vi "check_option.vi"(5 "Error generation (Error if missing)":T1, 7 "Attribute":T2={"Identifier"="", "Descriptive Name"="", "Data Type"=enum."Integer 32", "Command"="", "Access"=enum."Read/Write", "Range Table"="", "Read Callback"="", "Write Callback"="", "Supported Models"="", "Instrument Options"="", "Index"=0, "OPC Wait"=FALSE, "No Status Check"=FALSE, "Cache Only"=FALSE}, 8 "error in":errorcluster caption="error in (no error)", 11 "VISA resource name":refnum<visa-resource-name>) -> (0 "error out":errorcluster, 2 "Option installed":bool, 3 "VISA resource name out":refnum<visa-resource-name>)   [LabVIEW 2022 SP3, in "hmp4000_rsidr_core.lvlib"]
uses:
  hmp4000_rsidr_core.lvlib
  type_Attribute.ctl
  type_Attribute_Data_Type.ctl
  type_ReadWriteAccess.ctl
  type_InstrOptions_Error_GenMode.ctl
  type_Error_Codes.ctl
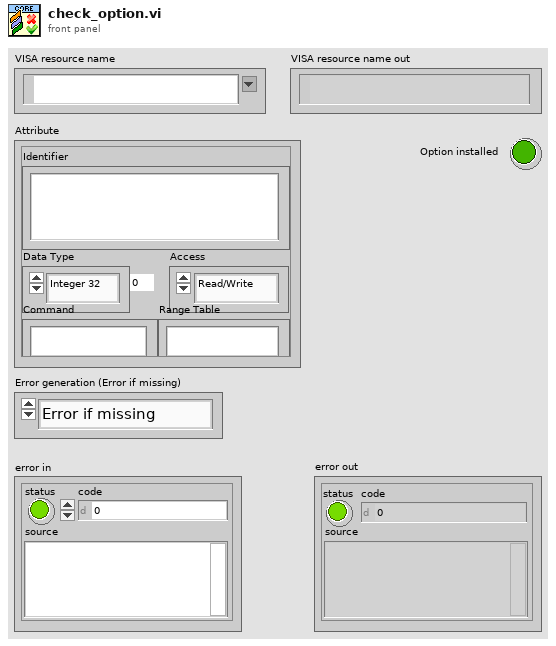
[diagram p1: front panel]
types:
  T1 = typedef "hmp4000_rsidr_core.lvlib/type_InstrOptions_Error_GenMode.ctl" = enum16{"Error if missing", "Error if present", "No error"}
  T2 = typedef "hmp4000_rsidr_core.lvlib/type_Attribute.ctl" = cluster{"Identifier":string, "Descriptive Name":string, "Data Type":T3, "Command":string, "Access":T4, "Range Table":string, "Read Callback":string, "Write Callback":string, "Supported Models":string, "Instrument Options":string, "Index":i32, "OPC Wait":bool, "No Status Check":bool, "Cache Only":bool}
  T3 = typedef "hmp4000_rsidr_core.lvlib/type_Attribute_Data_Type.ctl" = enum16{"Integer 32", "Double", "String", "Boolean", "None", "Integer 64", "RawString"}
  T4 = typedef "hmp4000_rsidr_core.lvlib/type_ReadWriteAccess.ctl" = enum16{"Read Only", "Write Only", "Read/Write"}
  T5 = typedef "hmp4000_rsidr_core.lvlib/type_Error_Codes.ctl" = enum16{"No_error", "VISA_err_ResourceNotFound", "VISA_err_Timeout", "VISA_warn_MoreDataAvailable", "RS_err_MissingCallback", "RS_err_InvalidAttribute", "RS_err_InvalidValue", "RS_err_UnknownResource", "RS_err_AlreadyInitialized", "RS_err_InstrumentStatus", "RS_err_BadRepCapName", "RS_err_TypesMismatch", "RS_err_ValueNotSupported", "RS_err_InvalidRngTable", "RS_err_IDqueryFail", "RS_err_UnexpResponse", "VISA_warn_ConfigNotLoaded", "RS_err_AttributeNotReadable", "RS_err_AttributeNotWritable", "RS_err_InstrumentType", "RS_err_InstrumentOption", "VISA_err_InvalidSize", "RS_err_ReliabilityIndicator", "VISA_warn_UnknownStatus", "VISA_warn_TermCharRead", "VISA_err_IO_error", "RS_err_FunctionNotSupported", "VISA_warn_QueueEmpty"}
  T6 = typedef "hmp4000_rsidr_core.lvlib/type_Session_Data.ctl" = cluster{"IDN string":string, "Instrument FW":string, "Instr type":string, "Instr type for err. msg.":string, "Installed Options":string[], "Ignore Error Messages":string, "Logging params":variant, "OPC Timeout":i32, "VISA Timeout":i32, "STB Poll VISA Timeout":i32, "Additional Flags":i32, "Wait Before Read":i32, "Wait Before Write":i32, "Option String Flags":i32, "IO Segment Size":i64, "VISA Access Mode":T7, "Interface Type":T8, "OPC Wait Mode":T9, "Bin Float Number  Format":T10, "Bin Integer Number Format":T11, "Simulate":bool, "VXIcapable":bool, "Duplicate Session":bool, "Add LF to Write":bool, "Logging":bool, "Fast Sweep":bool, "Query Instrument Status":bool, "Check Range":bool, "Check Options":bool}
  T7 = typedef "hmp4000_rsidr_core.lvlib/type_VisaAccessMode.ctl" = u16
  T8 = typedef "hmp4000_rsidr_core.lvlib/type_InterfaceType.ctl" = enum16{"Unknown", "GPIB", "VXI", "GPIB_VXI", "ASRL", "PXI", "TCPIP", "USB", "SOCKET"}
  T9 = typedef "hmp4000_rsidr_core.lvlib/type_OPC_Wait_Mode.ctl" = enum16{"STBpolling", "STBpollingSlow", "STBpollingSuperSlow", "ServiceRequest", "OPCquery"}
  T10 = typedef "hmp4000_rsidr_core.lvlib/type_Binary_Float_Number_Format.ctl" = enum16{"Float_4_Bytes_Swapped", "Float_4_Bytes", "Double_8_Bytes_Swapped", "Double_8_Bytes"}
  T11 = typedef "hmp4000_rsidr_core.lvlib/type_Binary_Integer_Number_Format.ctl" = enum16{"Int32_4_Bytes_Swapped", "Int32_4 Bytes", "Int16_2_Bytes_Swapped", "Int16_2_Bytes"}
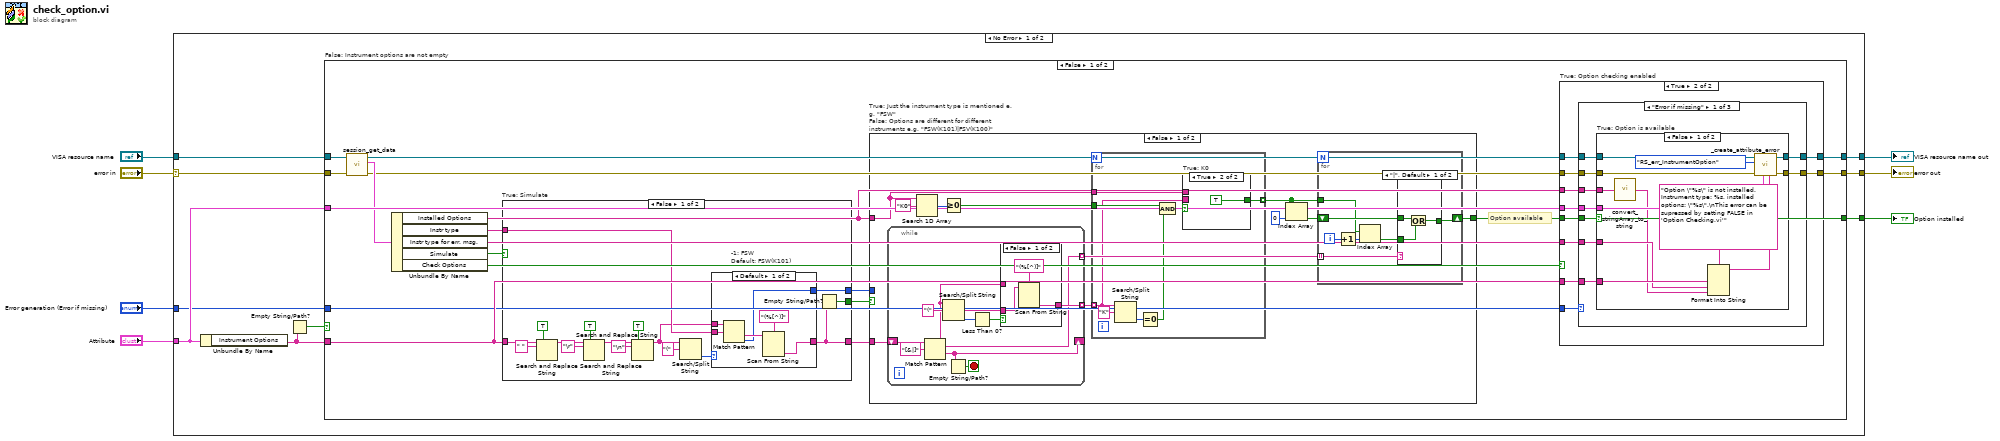
[diagram p0: block diagram]
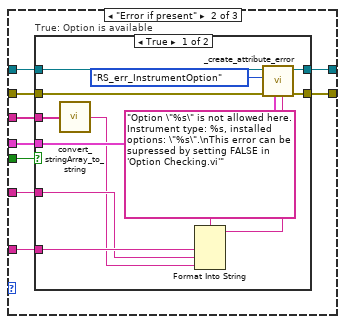
[diagram p4: hidden frame]
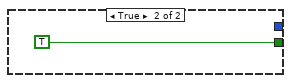
[diagram p8: hidden frame]
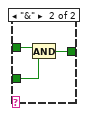
[diagram p9: hidden frame]
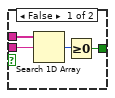
[diagram p10: hidden frame]
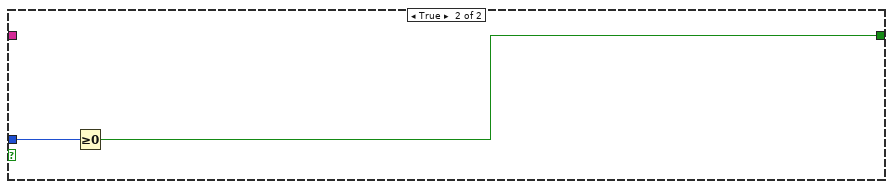
[diagram p12: hidden frame]
diagram:
  n1 = case shown="No Error" "error in" {
    selector: "error in" -> [w11 w176]
    tunnel: [w16 w176] -> w7
    tunnel: "Attribute" -> [w15 _]
    tunnel: "VISA resource name" -> [w10 w177]
    tunnel: [w13 w177] -> w4
    tunnel: "Error generation (Error if missing)" -> [w8 _]
    tunnel: [w9 _] -> w1
    frame No Error {
      n2 = Unbundle By Name(w15) -> ("Instrument Options"=w14:string)
      n3 = Empty String/Path?(string/path=w14) -> (empty?=w12:bool)
      n4 = case "False: Instrument options are not empty" shown="False" w12 {
        tunnel: w11 -> [w24 w175]
        tunnel: [w35 w175] -> w16
        tunnel: w14 -> [w32 _]
        tunnel: w15 -> [w33 _]
        tunnel: w10 -> [w23 w174]
        tunnel: [w27 w174] -> w13
        tunnel: [w17 _] -> w9
        tunnel: w8 -> [w19 _]
        frame False {
          # "Option available"
          n5 = call "session_get_data.vi"("error in"=w24, "VISA resource name"=w23) -> ("error out"=w21:errorcluster, "Session User Data out"=w22:T6, "VISA resource name out"=w20:refnum<visa-resource-name>)  [unwired: 6 in, 1 out]
          n6 = Unbundle By Name(w22) -> ("Installed Options"=w26:string[], "Instr type"=w34:string, "Instr type for err. msg."=w31:string, "Simulate"=w25:bool, "Check Options"=w18:bool)
          n7 = case "True: Simulate" shown="False" w25 {
            tunnel: w34 -> [w111 _]
            tunnel: w32 -> [w110 _]
            tunnel: [w98 _] -> w30
            tunnel: [w96 TRUE] -> w29
            tunnel: [w97 _] -> w28
            frame False {
              n8 = Search and Replace String(replace all?=TRUE ("replace all? (F)"), input string=w110, search string=" ") -> (result string=w103:string)  [unwired: 5 in, 3 out]
              n9 = Search and Replace String(replace all?=TRUE ("replace all? (F)"), input string=w103, search string="\r") -> (result string=w102:string)  [unwired: 5 in, 3 out]
              n10 = Search and Replace String(replace all?=TRUE ("replace all? (F)"), input string=w102, search string="\n") -> (result string=w99:string)  [unwired: 5 in, 3 out]
              n11 = Search/Split String(string=w99, search string/char (-)="(") -> (offset of match=w100:i32)  [unwired: 1 in, 2 out]
              n12 = case "-1: FSW\nDefault: FSW(K101)" shown="Default" w100 {
                tunnel: w99 -> [w117 w118]
                tunnel: [w113 w118] -> w97
                tunnel: w111 -> [w116 _]
                tunnel: [w112 _] -> w98
                frame Default {
                  n13 = Match Pattern(string=w117, regular expression=w116) -> (after substring=w115:string, offset past match=w112:i32)  [unwired: 1 in, 2 out]
                  n14 = Scan From String(format string="(%[^)]", input string=w115) -> (output 1=w113:string)  [unwired: 3 in, 3 out]
                }
                frame -1 {
                }
              }
              n15 = Empty String/Path?(string/path=w97) -> (empty?=w96:bool)
            }
            frame True {
            }
          }
          n16 = case "True: Just the instrument type is mentioned e.g. \"FSW\"\nFalse: Options are different for different instruments e.g. \"FSW(K101)|FSV(K100)\"" shown="False" w29 {
            tunnel: [w127 w172] -> w17
            tunnel: w28 -> [w126 _]
            tunnel: w26 -> [w124 _]
            tunnel: w30 -> [_ w173]
            frame False {
              n17 = while {
                shift-right: [w157] -> _
                shift-left: w126 -> [w167]
                tunnel: [w160] -> w120 mode=indexing
                tunnel: [w159] -> w130 mode=indexing
                stop <- w165 stop-if-true
                n18 = Match Pattern(string=w167, regular expression="[&|]") -> (before substring=w158:string, match substring=w159:string, after substring=w157:string)  [unwired: 1 in, 1 out]
                n19 = Search/Split String(string=w158, search string/char (-)="(") -> (match + rest of string=w163:string, offset of match=w162:i32)  [unwired: 1 in, 1 out]
                n20 = Empty String/Path?(string/path=w157) -> (empty?=w165:bool)
                n21 = Less Than 0?(x=w162) -> (x < 0?=w161:bool)
                n22 = case shown="False" w161 {
                  tunnel: w163 -> [w168 _]
                  tunnel: [w169 w171] -> w160
                  tunnel: w158 -> [_ w171]
                  frame False {
                    n23 = Scan From String(format string="(%[^)]", input string=w168) -> (output 1=w169:string)  [unwired: 3 in, 3 out]
                  }
                  frame True {
                  }
                }
              }
              n24 = Search 1D Array(1D array=w124, element="K0") -> (index of element=w122:i32)  [unwired: 1 in]
              n25 = Greater Or Equal To 0?(x=w122) -> (x >= 0?=w121:bool)
              n26 = for {
                tunnel: w124 -> [w151]
                tunnel: [w150] -> w125 mode=indexing
                tunnel: w121 -> [w146]
                tunnel: w120 -> [w145] mode=indexing
                n27 = Search/Split String(string=w145, search string/char (-)="K") -> (offset of match=w148:i32)  [unwired: 1 in, 2 out]
                n28 = Equal To 0?(x=w148) -> (x = 0?=w147:bool)
                n29 = Compound Arithmetic op=AND(w146, w147) -> (w144:bool)
                n30 = case "True: K0" shown="True" w144 {
                  tunnel: w151 -> [w155 _]
                  tunnel: [w153 TRUE] -> w150
                  tunnel: w145 -> [w152 _]
                  frame False {
                    n31 = Search 1D Array(1D array=w155, element=w152) -> (index of element=w154:i32)  [unwired: 1 in]
                    n32 = Greater Or Equal To 0?(x=w154) -> (x >= 0?=w153:bool)
                  }
                  frame True {
                  }
                }
              }
              n33 = Index Array(array=w125, index=0) -> (element=w129:bool)
              n34 = for {
                tunnel: w130 -> [w131] mode=indexing
                tunnel: w125 -> [w135]
                shift-right: [w136] -> w127
                shift-left: w129 -> [w137]
                i -> [w133]
                n35 = Increment(x=w133) -> (x+1=w134:i32)
                n36 = Index Array(array=w135, index=w134) -> (element=w132:bool)
                n37 = case shown="\"|\", Default" w131 {
                  tunnel: w137 -> [w139 w143]
                  tunnel: [w140 w142] -> w136
                  tunnel: w132 -> [w138 w141]
                  frame "|", Default {
                    n38 = Or(x=w139, y=w138) -> (x .or. y?=w140:bool)
                  }
                  frame "&" {
                    n39 = And(x=w143, y=w141) -> (x .and. y?=w142:bool)
                  }
                }
              }
            }
            frame True {
              n40 = Greater Or Equal To 0?(x=w173) -> (x >= 0?=w172:bool)
            }
          }
          n41 = case "True: Option checking enabled" shown="True" w18 {
            tunnel: [w37 w47] -> w35
            tunnel: w33 -> [_ w46]
            tunnel: w32 -> [_ w45]
            tunnel: w31 -> [_ w44]
            tunnel: [w36 w43] -> w27
            tunnel: w26 -> [_ w42]
            tunnel: w21 -> [w37 w41]
            tunnel: w20 -> [w36 w40]
            tunnel: w19 -> [_ w39]
            tunnel: w17 -> [_ w38]
            frame False {
            }
            frame True {
              n42 = case shown="\"Error if missing\"" w39 {
                tunnel: [w56 w79 w95] -> w47
                tunnel: w46 -> [w55 w78 _]
                tunnel: w45 -> [w54 w77 _]
                tunnel: w44 -> [w53 w76 _]
                tunnel: [w52 w75 w94] -> w43
                tunnel: w42 -> [w51 w74 _]
                tunnel: w41 -> [w50 w73 w95]
                tunnel: w40 -> [w49 w72 w94]
                tunnel: w38 -> [w48 w71 _]
                frame "Error if missing" {
                  n43 = case "True: Option is available" shown="False" w48 {
                    tunnel: w50 -> [w67 w70]
                    tunnel: [w68 w70] -> w56
                    tunnel: w55 -> [w64 _]
                    tunnel: w54 -> [w66 _]
                    tunnel: w53 -> [w58 _]
                    tunnel: w49 -> [w61 w69]
                    tunnel: [w60 w69] -> w52
                    tunnel: w51 -> [w59 _]
                    frame False {
                      n44 = call "convert_stringArray_to_string.vi"("string array in"=w59) -> ("string out"=w57:string)  [unwired: 4 in]
                      n45 = Format Into String(format string="Option \"%s\" is not installed. Instrument type: %s, installed options: \"%s\".\nThis error can be supressed by setting FALSE in 'Option Checking.vi'" ("string"), w66, w58, w57) -> (resulting string=w63:string)  [unwired: 2 in, 1 out]
                      n46 = call "_create_attribute_error.vi"("Error Elaboration (\"\")"=w63, "Attribute"=w64, "error in"=w67, "Error Enum in"=type_Error_Codes."RS_err_InstrumentOption" ("Error Enum in (from err to recompose)"), "VISA resource name"=w61) -> ("error out"=w68:errorcluster, "VISA resource name out"=w60:refnum<visa-resource-name>)  [unwired: 5 in]
                    }
                    frame True {
                    }
                  }
                }
                frame "Error if present" {
                  n47 = case "True: Option is available" shown="True" w71 {
                    tunnel: w73 -> [w90 w93]
                    tunnel: [w91 w93] -> w79
                    tunnel: w78 -> [w87 _]
                    tunnel: w77 -> [w89 _]
                    tunnel: w76 -> [w81 _]
                    tunnel: w72 -> [w84 w92]
                    tunnel: [w83 w92] -> w75
                    tunnel: w74 -> [w82 _]
                    frame True {
                      n48 = call "convert_stringArray_to_string.vi"("string array in"=w82) -> ("string out"=w80:string)  [unwired: 4 in]
                      n49 = Format Into String(format string="Option \"%s\" is not allowed here. Instrument type: %s, installed options: \"%s\".\nThis error can be supressed by setting FALSE in 'Option Checking.vi'" ("string"), w89, w81, w80) -> (resulting string=w86:string)  [unwired: 2 in, 1 out]
                      n50 = call "_create_attribute_error.vi"("Error Elaboration (\"\")"=w86, "Attribute"=w87, "error in"=w90, "Error Enum in"=type_Error_Codes."RS_err_InstrumentOption" ("Error Enum in (from err to recompose)"), "VISA resource name"=w84) -> ("error out"=w91:errorcluster, "VISA resource name out"=w83:refnum<visa-resource-name>)  [unwired: 5 in]
                    }
                    frame False {
                    }
                  }
                }
                frame "No error" {
                }
              }
            }
          }
        }
        frame True {
        }
      }
    }
    frame Error {
    }
  }
  "error out" <- w7
  "VISA resource name out" <- w4
  "Option installed" <- w1
